vi "適應性控制DAQmx API(實際控制).vi"() -> ()   [LabVIEW 2010]
uses:
  <vilib>/DAQmx/read.llb/DAQmx Read (Analog DBL 1Chan 1Samp).vi
  <vilib>/DAQmx/create/channels.llb/DAQmx Create Channel (AI-Voltage-Basic).vi
  <vilib>/DAQmx/configure/timing.llb/DAQmx Timing (Sample Clock).vi
  <vilib>/daqmx/miscellaneous.llb/DAQmx Fill In Error Info.vi
panel:
  in  "timeout 2":dbl=10.0 format="%0.2f"
  in  "physical channels 2":tag
  in  "timeout":dbl=10.0 format="%0.2f"
  in  "physical channels":tag
  in  "number of samples":i32=100
  out "while 每次運行時間":u32
  in  "rate":dbl=1000.0
  out "收斂時間(s)":dbl
  out "收斂燈":bool
  in  "ERR誤差低於多少V亮燈":dbl=0.05
  out "ERR message":string=" INSTRUCTIONS:\r\rNormal Use:  When using subVIs that incorporate the error in/error out (or error I/O) structure, place this handler where you want to inform the user of an error, typically at the end of the I/O data path, as the last action of the program.  If the error in error? is ERROR, the handler creates a message describing the error and its source.  If the type of dialog = 1 (default), the message is displayed to the user, who can only acknowedge it.  If the type = 2, the user can acknowledge the message or abort execution; aborting a program with active I/O is not recommended.  If the type = 0, no message is displayed; this is used to process the error programmatically, and the error out cluster elements are wired to individual terminals for that reason.  \r\rOther Use:\n\r\nlocal testing.  To test the error code of a subVI or function that does not have the error I/O structure, you can wire its error code and a source string to the local error code and error source inputs.  If error in error? indicates no error and error code is not equal to 0, the local code and source are substituted for the error in values, and error? is set TRUE (ERROR)."
  out "理想系統與FIR輸出":cluster{dbl, dbl}(graph)
  out "system輸出":dbl
  out "input_x(t)":dbl(graph)
  out "ERR":dbl(graph)
  out "權重函數向量":dbl[](array[numeric])
  in  "order":i32=8
  out "LMS":dbl[](graph)
  out "FIR輸出":dbl
  in  "Stop Button":bool
  in  "u(收斂係數)":dbl=0.005
  # "A0:模擬輸入 pulse_output 2"
  # "A1:理想系統 pulse_output 1"
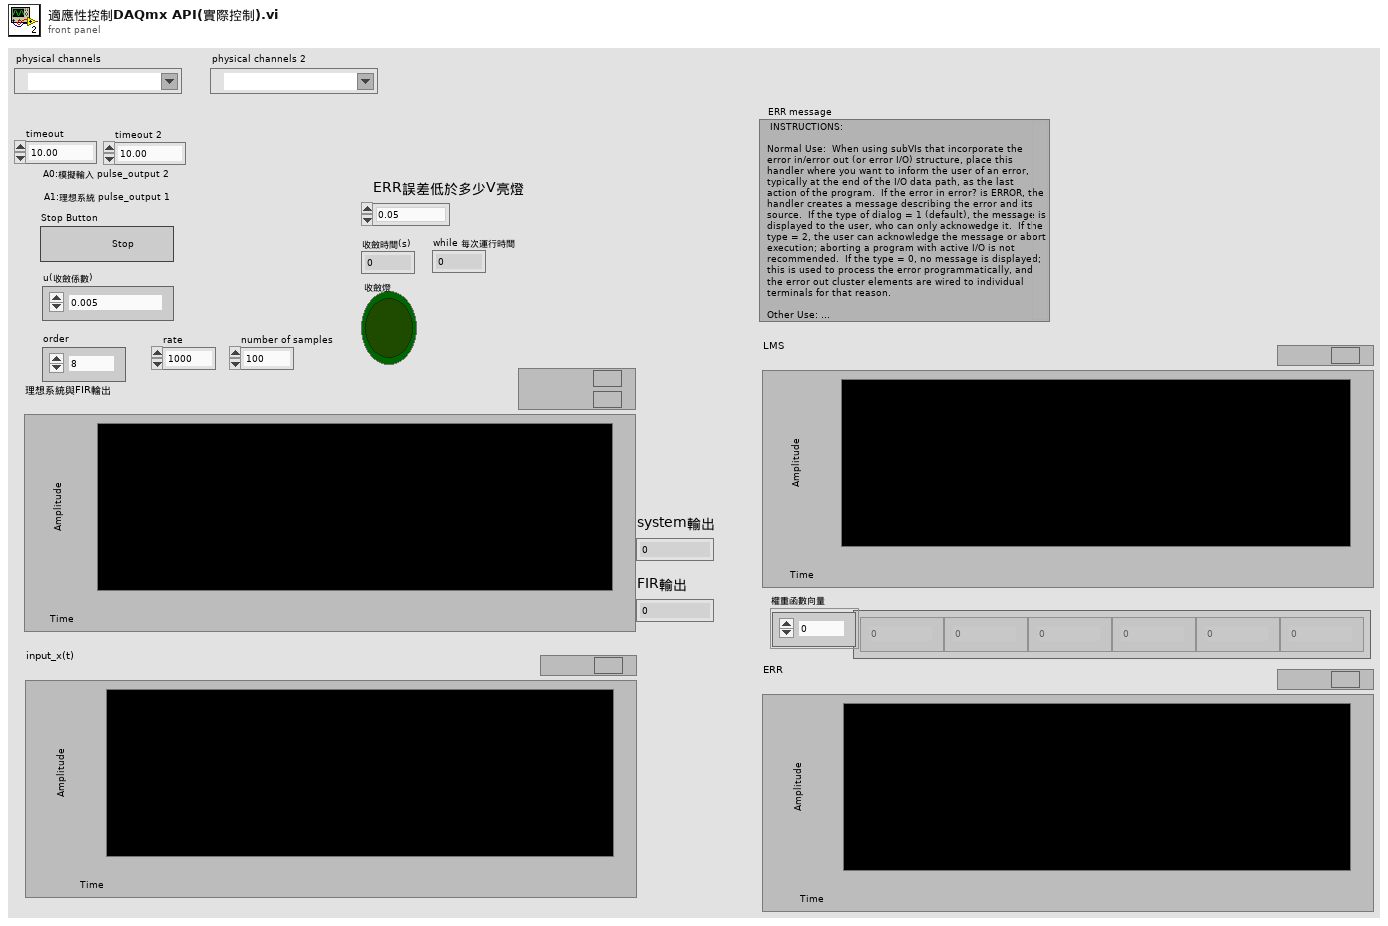
[diagram p1: front panel]
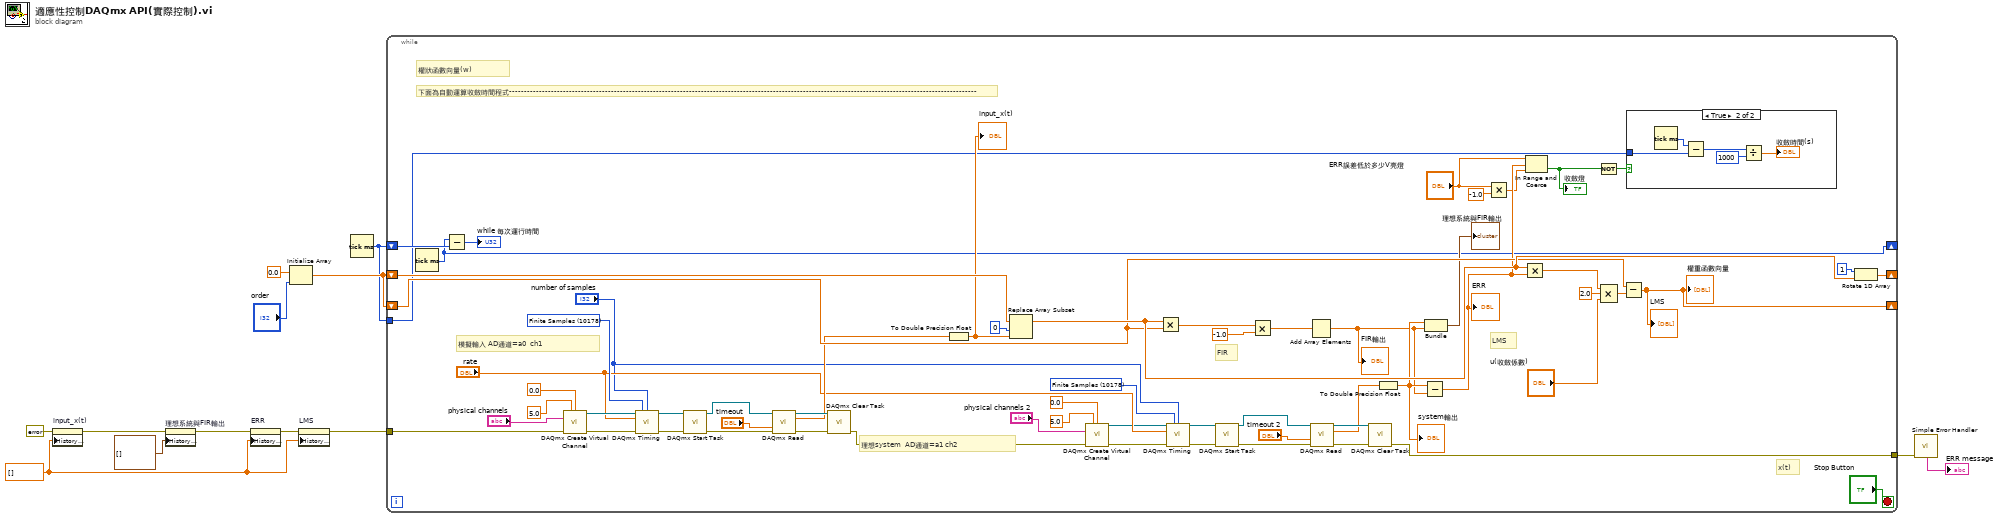
[diagram p0: block diagram]
diagram:
  w9 = dbl[] [] ("History Data")
  n1 = property on="input_x(t)" class="WFChart (strict)"(error in=errorcluster {"status"=FALSE, "code"=0, "source"=""} ("error constant"), "History Data"=w9) -> (error out=w6:errorcluster)  [unwired: 1 in, 1 out]
  n2 = property on="理想系統與FIR輸出" class="WFChart (strict)"(error in=w6, "History Data"=cluster{dbl, dbl}[] []) -> (error out=w5:errorcluster)  [unwired: 1 in, 1 out]
  n3 = property on="ERR" class="WFChart (strict)"(error in=w5, "History Data"=w9) -> (error out=w7:errorcluster)  [unwired: 1 in, 1 out]
  n4 = Initialize Array "Initialize Array"(0.0 ("element"), "order") -> (w11:dbl[])
  n5 = property on="LMS" class="WFChart (strict)"(error in=w7, "History Data"=w9) -> (error out=w8:errorcluster)  [unwired: 1 in, 1 out]
  n6 = Tick Count (ms)() -> (millisecond timer value=w1:u32)
  n7 = while {
    shift-right: [w66] -> _
    shift-left: w11 -> [w65]
    shift-right: [w62] -> _
    shift-left: w11 -> [w61]
    tunnel: w8 -> [w32]
    tunnel: [w16] -> w3
    shift-right: [w48] -> _
    shift-left: w1 -> [w50]
    tunnel: w1 -> [w49]
    stop <- "Stop Button" stop-if-true
    w26 = 10178 items=["Finite Samples"=10178, "Continuous Samples"=10123, "Hardware Timed Single Point"=12522] ("sample mode")
    w35 = 10178 items=["Finite Samples"=10178, "Continuous Samples"=10123, "Hardware Timed Single Point"=12522] ("sample mode")
    # "下面為自動運算收斂時間程式------------------------------------------------------------------------------------------------------------------------------------------------------------"
    # "LMS"
    # "FIR"
    # "模擬輸入 AD通道=a0  ch1"
    # "權狀函數向量(w)"
    # "x(t)"
    # "理想system  AD通道=a1 ch2"
    n8 = Tick Count (ms)() -> (millisecond timer value=w48:u32)
    n9 = Subtract(x=w48, y=w50) -> (x-y=→"while 每次運行時間":u32)
    n10 = call-poly <vilib>:"DAQmx Create Virtual Channel.vi"("maximum value"=5.0, "minimum value"=0.0, "physical channels"="physical channels", "error in"=w32) -> ("task out"=w44:refnum<k21>, "error out"=w45:errorcluster)  [unwired: 10 in]
    n11 = call-poly <vilib>:"DAQmx Timing.vi"("task/channels in"=w44, "sample mode"=w35, "samples per channel"="number of samples", "rate"="rate", "error in"=w45) -> ("task out"=w42:refnum<k21>, "error out"=w43:errorcluster)  [unwired: 9 in]
    n12 = call <vilib>:"DAQmx Start Task.vi"("task/channels in"=w42, "error in"=w43) -> ("task out"=w40:refnum<k21>, "error out"=w41:errorcluster)  [unwired: 12 in]
    n13 = call-poly <vilib>:"DAQmx Read.vi"("task/channels in"=w40, "timeout"="timeout", "error in"=w41) -> ("task out"=w38:refnum<k21>, "data"=w33:dbl, "error out"=w39:errorcluster)  [unwired: 10 in]
    n14 = call <vilib>:"DAQmx Clear Task.vi"("task in"=w38, "error in"=w39) -> ("error out"=w15:errorcluster)  [unwired: 13 in]
    n15 = To Double Precision Float(number=w33) -> (double precision float=w60:dbl)
    "input_x(t)" <- w60
    n16 = Replace Array Subset "Replace Array Subset"(array=w65, new element=w60, index=0) -> (w63:dbl[])
    n17 = call-poly <vilib>:"DAQmx Create Virtual Channel.vi"("maximum value"=5.0, "minimum value"=0.0, "physical channels"="physical channels 2", "error in"=w15) -> ("task out"=w27:refnum<k21>, "error out"=w22:errorcluster)  [unwired: 10 in]
    n18 = Multiply(x=w63, y=w61) -> (x*y=w75:dbl[])
    n19 = call-poly <vilib>:"DAQmx Timing.vi"("task/channels in"=w27, "sample mode"=w26, "samples per channel"="number of samples", "rate"="rate", "error in"=w22) -> ("task out"=w25:refnum<k21>, "error out"=w21:errorcluster)  [unwired: 9 in]
    n20 = call <vilib>:"DAQmx Start Task.vi"("task/channels in"=w25, "error in"=w21) -> ("task out"=w24:refnum<k21>, "error out"=w20:errorcluster)  [unwired: 12 in]
    n21 = Multiply(x=w75, y=-1.0) -> (x*y=w68:dbl[])
    n22 = Add Array Elements(numeric array=w68) -> (sum=w58:dbl)
    "FIR輸出" <- w58
    n23 = call-poly <vilib>:"DAQmx Read.vi"("task/channels in"=w24, "timeout"="timeout 2", "error in"=w20) -> ("task out"=w23:refnum<k21>, "data"=w18:dbl, "error out"=w19:errorcluster)  [unwired: 10 in]
    n24 = call <vilib>:"DAQmx Clear Task.vi"("task in"=w23, "error in"=w19) -> ("error out"=w16:errorcluster)  [unwired: 13 in]
    n25 = To Double Precision Float(number=w18) -> (double precision float=w59:dbl)
    "system輸出" <- w59
    n26 = Subtract(x=w59, y=w58) -> (x-y=w56:dbl)
    "ERR" <- w56
    n27 = Bundle(w59, w58) -> (→"理想系統與FIR輸出":cluster{dbl, dbl})  [unwired: 1 in]
    n28 = Multiply(x="ERR誤差低於多少V亮燈", y=-1.0) -> (x*y=w55:dbl)
    n29 = Multiply(x=w63, y=w56) -> (x*y=w73:dbl[])
    n30 = In Range and Coerce(upper limit="ERR誤差低於多少V亮燈", x=w56, lower limit=w55) -> (In Range?=w51:bool)  [unwired: 1 out]
    "收斂燈" <- w51
    n31 = Not(x=w51) -> (.not. x?=w52:bool)
    n32 = Compound Arithmetic op=MULTIPLY(w73, 2.0 ("value"), "u(收斂係數)") -> (w70:dbl[])
    n33 = Subtract(x=w61, y=w70) -> (x-y=w62:dbl[])
    "LMS" <- w62
    "權重函數向量" <- w62
    n34 = case shown="True" w52 {
      tunnel: w49 -> [_ w79]
      frame False {
      }
      frame True {
        n35 = Tick Count (ms)() -> (millisecond timer value=w80:u32)
        n36 = Subtract(x=w80, y=w79) -> (x-y=w78:u32)
        n37 = Divide(x=w78, y=u32 1000) -> (x/y=→"收斂時間(s)":dbl)
      }
    }
    n38 = Rotate 1D Array(1:w63, 2:1 ("n")) -> (0:w66:dbl[])
  }
  n39 = call <vilib>:"Simple Error Handler.vi"("error in (no error)"=w3) -> ("message"=→"ERR message":string)  [unwired: 4 in, 4 out]
